vi "230427_Database_read.vi"() -> ()   [LabVIEW 2022 SP3]
uses:
  <vilib>/addons/database/Connection.llb/DB Tools Open Connec (Path).vi
  <vilib>/addons/database/_DB Variant To Data/Database Variant To Data.xnode
  <vilib>/addons/database/NI_Database_API.lvlib
panel:
  out "data":string[][](array[string])
  in  "table":string
  in  "connection information":path
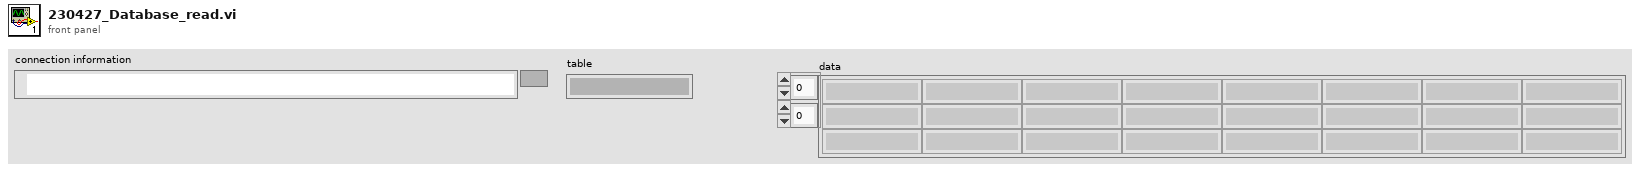
[diagram p1: front panel]
types:
  T1 = typedef "NI_Database_API.lvlib/Conn ObjectReference.ctl" = refnum<k1>
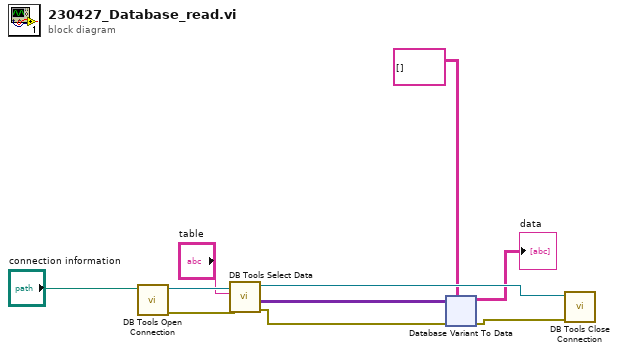
[diagram p0: block diagram]
diagram:
  n1 = call-poly <vilib>:"DB Tools Open Connection.vi"("connection information"="connection information") -> ("error out"=w8:errorcluster, "connection reference"=w9:T1)  [unwired: 7 in]
  n2 = call <vilib>:"DB Tools Select Data.vi"("error in (no error)"=w8, "table"="table", "connection reference"=w9) -> ("error out"=w5:errorcluster, "data"=w6:variant[][], "connection reference out"=w3:T1)  [unwired: 3 in]
  n3 = xnode "Database Variant To Data"("database variant"=w6, "error in (no error)"=w5, "type"=string[][] []) -> ("data"=→"data":string[][], "error out"=w4:errorcluster)
  n4 = call <vilib>:"DB Tools Close Connection.vi"("error in (no error)"=w4, "connection reference"=w3) -> ()  [unwired: 5 in, 1 out]
